vi "Exposure-Config.vi"(0 "Exposure parameters":T27, 1 "Expt State":T3, 5 "Filter options":cluster{"InvFilt":bool, "Brickwall":bool}, 7 "Sampling rate (Hz)":dbl, 9 "Buffer length (s)":dbl, 11 "error in (no error)":errorcluster, 12 "Options":T2={"Tracking"={"Tolerance (dB)"=0.25, "T (s)"=3.0}, "Seeds"={"Left"=0, "Right"=0}}) -> (2 "SPL Log":cluster{dbl, "Buffer length (s)":dbl, dbl[][]}, 3 "Runtime":T4, 4 "AO Channels":i32[](array[numeric]), 6 "stimulus":T5[](array[typedef]) {"Filter"."IIR Filter Cluster"."Forward Coefficients" format="%.4f"; "Filter"."IIR Filter Cluster"."Reverse Coefficients" format="%.4f"}, 8 "InvFilt":T1[](array[typedef]), 10 "Npts":i32, 13 "Max SPL History":dbl[][](array[numeric]), 14 "Num Buffers":i32, 15 "error out":errorcluster)   [LabVIEW 2020]
uses:
  Typedefs/Exposure Parameters.ctl
  epl-vi-lib/Signal Synthesis VIs/Controls/Stimulus Channel XCtl/Stimulus Channel Data.ctl
  epl-vi-lib/Signal Synthesis VIs/Controls/Waveform XCtl/Waveform Data.ctl
  epl-vi-lib/Signal Synthesis VIs/Controls/Waveform XCtl/Waveform Enum.ctl
  epl-vi-lib/Signal Synthesis VIs/Waveform VIs/Tone VIs/Tone Params.ctl
  epl-vi-lib/Signal Synthesis VIs/Waveform VIs/Pulse Train VIs/Pulse Train Params.ctl
  epl-vi-lib/Signal Synthesis VIs/Waveform VIs/Pulse Train VIs/Pulse Polarity.ctl
  epl-vi-lib/Signal Synthesis VIs/Waveform VIs/Pulse Train VIs/PT-Continuous State.ctl
  epl-vi-lib/Signal Synthesis VIs/Waveform VIs/Noise VIs/Noise Params.ctl
  epl-vi-lib/Signal Synthesis VIs/Waveform VIs/File VIs/StimFile-Params.ctl
  epl-vi-lib/Signal Synthesis VIs/Waveform VIs/FM Sweep VIs/FM Sweep Params.ctl
  epl-vi-lib/Signal Synthesis VIs/Waveform VIs/Chirp Train VIs/Chirp Train.ctl
  epl-vi-lib/Signal Synthesis VIs/Waveform VIs/Chirp Train VIs/Chirp Train Params.ctl
  epl-vi-lib/Signal Synthesis VIs/Waveform VIs/Complex Tone VIs/CT-Params.ctl
  epl-vi-lib/Signal Synthesis VIs/Waveform VIs/Complex Tone VIs/CT-Phase Enum.ctl
  epl-vi-lib/Signal Synthesis VIs/Waveform VIs/Complex Tone VIs/CT-Runtime Data.ctl
  epl-vi-lib/Signal Synthesis VIs/Waveform VIs/Moving Ripple VIs/Moving Ripple.ctl
  epl-vi-lib/Signal Synthesis VIs/Waveform VIs/Moving Ripple VIs/Moving Ripple.Params.ctl
  epl-vi-lib/Signal Synthesis VIs/Waveform VIs/Moving Ripple VIs/Moving Ripple.Data.ctl
  epl-vi-lib/Signal Synthesis VIs/Controls/Filter XCtl/Filter Data.ctl
  epl-vi-lib/Signal Synthesis VIs/Controls/Gate XCtl/Gate Data.ctl
  epl-vi-lib/Signal Synthesis VIs/Controls/Level XCtl/Level Data.ctl
  epl-vi-lib/Signal Synthesis VIs/Controls/Level XCtl/Level Units.ctl
  Typedefs/Exposure-Runtime Data.ctl
  CFTS Main Panel SubVIs/CFTS-Experiment State.ctl
  Typedefs/Exposure-Options.ctl
  Typedefs/Exposure-Inverse Filter Runtime.ctl
  epl-vi-lib/Connection VIs/Type Defs/Output sources.ctl
  epl-vi-lib/Connection VIs/Type Defs/Input sources.ctl
  epl-vi-lib/Utility VIs/Array Manipulation VIs/Sort and Index (I32).vi
  epl-vi-lib/Signal Synthesis VIs/Top Level VIs/Stimulus-Set Level (array).vi
  epl-vi-lib/Signal Synthesis VIs/Controls/Filter XCtl/Filter XCtl.xctl
  epl-vi-lib/Signal Synthesis VIs/Controls/Level XCtl/Level XCtl.xctl
  epl-vi-lib/Signal Synthesis VIs/Controls/Gate XCtl/Gate Control.xctl
  epl-vi-lib/Signal Synthesis VIs/Controls/Waveform XCtl/Waveform XCtl.xctl
  epl-vi-lib/Signal Synthesis VIs/Controls/Stimulus Channel XCtl/Stimulus Channel.xctl
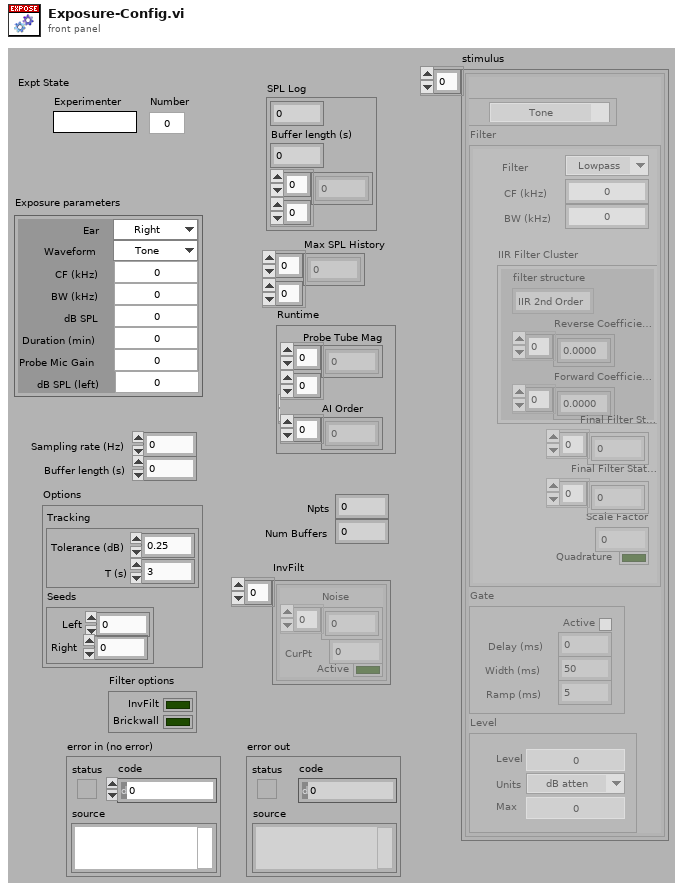
[diagram p1: front panel]
types:
  T1 = typedef "Exposure-Inverse Filter Runtime.ctl" = cluster{"Noise":dbl[], "CurPt":i32, "Active":bool}
  T2 = typedef "Exposure-Options.ctl" = cluster{"Tracking":cluster{"Tolerance (dB)":dbl, "T (s)":dbl}, "Seeds":cluster{"Left":i32, "Right":i32}}
  T3 = typedef "CFTS-Experiment State.ctl" = cluster{"Experimenter":string, "Number":u32, "Right":string, "Left":string, "Data Folder":path, "State File":path, "Version Info":string, "End Exposure Time":dbl, "Exposure Duration":string, "Run #":cluster{"CAP":i16, "ABR":i16, "DP":i16, "VsEP":i16, "MeasSeq":i16, "SubSeq":i16, "SFOAE":i16}}
  T4 = typedef "Exposure-Runtime Data.ctl" = cluster{"Probe Tube Mag":dbl[][], "AI Order":i32[]}
  T5 = typedef "Stimulus Channel.xctl/Stimulus Channel Data.ctl" = cluster{"Waveform":T6, "Filter":T23, "Gate":T24, "Level":T25}
  T6 = typedef "Waveform XCtl.xctl/Waveform Data.ctl" = cluster{"Type":T7, "Tone":T8, "Pulse Train":T9, "Noise":T12, "File":T13, "FMSweep":T14, "Chirp Train":T15, "Complex Tone":cluster{"Params":T17, "Data":T19}, "Moving Ripple":T20}
  T7 = typedef "Waveform Enum.ctl" = enum16{"OFF", "Tone", "Noise", "Pulse Train", "File", "FM Sweep", "Chirp Train", "Complex Tone", "FM Tone", "Moving Ripple"}
  T8 = typedef "Tone Params.ctl" = cluster{"Frequency (kHz)":dbl, "Last Freq":dbl, "Last Phase":dbl}
  T9 = typedef "Pulse Train Params.ctl" = cluster{"Pulse width (us)":dbl, "Pulse rate (Hz)":dbl, "Gap (ms)":dbl, "Polarity":T10, "PT State":T11, "Asynch":bool}
  T10 = typedef "Pulse Polarity.ctl" = enum16{"POS", "NEG", "POS-NEG", "NEG-POS"}
  T11 = typedef "PT-Continuous State.ctl" = cluster{"Template":dbl[], "Nperiod":i32, "Index":i32, "Pulse Rate (Hz)":dbl, "Phase (cycles)":dbl, "Noff":i32}
  T12 = typedef "Noise Params.ctl" = cluster{"InvFilt":bool, "Noise":dbl[], "CurPt":i32, "Aweight":bool, "Seed":i32, "afile":path}
  T13 = typedef "StimFile-Params.ctl" = cluster{"Filename":path, "Signal":dbl[], "Channel":i32, "stream":bool, "offset":i32, "nreps":i32, "loops":i32, "Randomize":bool, "order":i32[], "Seed":i32, "Tokens":i32}
  T14 = typedef "FM Sweep Params.ctl" = cluster{"Rate (oct/s)":dbl, "Fmin (Hz)":dbl, "Fmax (Hz)":dbl, "Ramp (ms)":dbl, "Linear":bool}
  T15 = typedef "Chirp Train.ctl" = cluster{"Params":T16, "Data":cluster{"WF":dbl[]}}
  T16 = typedef "Chirp Train Params.ctl" = cluster{"Fmin (kHz)":dbl, "Fmax (kHz)":dbl, "Compensate":bool, "Duration (ms)":dbl}
  T17 = typedef "CT-Params.ctl" = cluster{"F0 (Hz)":dbl, "Band":cluster{"Flow (Hz)":dbl, "Fhigh (Hz)":dbl}, "Phase":T18, "Min F0 (Hz)":dbl, "Max F0 (Hz)":dbl, "ContinRandPhase":bool, "Max peak factor":dbl, "Max mod depth":dbl, "MinHarmNum":i32, "MaxHarmNum":i32, "Level Mode":enum16{"per component", "overall rms"}, "% jitter":dbl}
  T18 = typedef "CT-Phase Enum.ctl" = enum16{"Cosine", "Random", "Alternating"}
  T19 = typedef "CT-Runtime Data.ctl" = cluster{"Ncomp":i32, "MinHarm":i32, "Phase":dbl[], "Amplitude":dbl[], "Npts/frame":i32, "Last F0":dbl, "Fmin":dbl, "Fmax":dbl, "Lslope":dbl, "randphase":bool, "overall rms":bool, "fmult":dbl[], "jittered":bool}
  T20 = typedef "Moving Ripple.ctl" = cluster{"Params":T21, "Data":T22}
  T21 = typedef "Moving Ripple.Params.ctl" = cluster{"Fmin":dbl, "Fmax":dbl, "Density":dbl, "Velocity":dbl, "Depth":dbl, "Phase":dbl, "Comp/oct":i32}
  T22 = typedef "Moving Ripple.Data.ctl" = cluster{"Freq":dbl[], "A":dbl[], "phase":dbl[], "Phase":dbl}
  T23 = typedef "Filter XCtl.xctl/Filter Data.ctl" = cluster{"CF (kHz)":dbl, "BW (kHz)":dbl, "IIR Filter Cluster":cluster{"filter structure":enum32{"IIR 2nd Order", "IIR 4th Order"}, "Reverse Coefficients":dbl[], "Forward Coefficients":dbl[]}, "Final Filter State":dbl[], "Scale Factor":dbl, "Final Filter State 2":dbl[], "Quadrature":bool, "Type":enum16{"Lowpass", "Highpass", "Bandpass", "Bandstop", "OFF"}}
  T24 = typedef "Gate Control.xctl/Gate Data.ctl" = cluster{"Active":bool, "Delay (ms)":dbl, "Width (ms)":dbl, "Ramp (ms)":dbl}
  T25 = typedef "Level XCtl.xctl/Level Data.ctl" = cluster{"Level":dbl, "Units":T26, "Max":dbl, "Multiplier":dbl, "Cal File":path, "Cal":cluster{"Freq (Hz)":dbl[], "Mag (dB SPL)":dbl[], "Phase (deg)":dbl[]}}
  T26 = typedef "Level Units.ctl" = enum16{"dB atten", "dB SPL", "dB re 1 Vrms", "dB V/Hz½", "mW", "dB HL", "Volts", "dB mW"}
  T27 = typedef "Exposure Parameters.ctl" = cluster{"Probe Mic Gain":dbl, "Waveform":enum16{"Tone", "Noise"}, "CF (kHz)":dbl, "BW (kHz)":dbl, "Ear":enum16{"Right", "Left", "Binaural"}, "Duration (min)":dbl, "dB SPL":dbl, "dB SPL (left)":dbl}
  T28 = typedef "Input sources.ctl" = u16
  T29 = typedef "Output sources.ctl" = u16
  T30 = cluster{"Waveform":T6, "Filter":T23, "Gate":T24, "Level":T25}[]
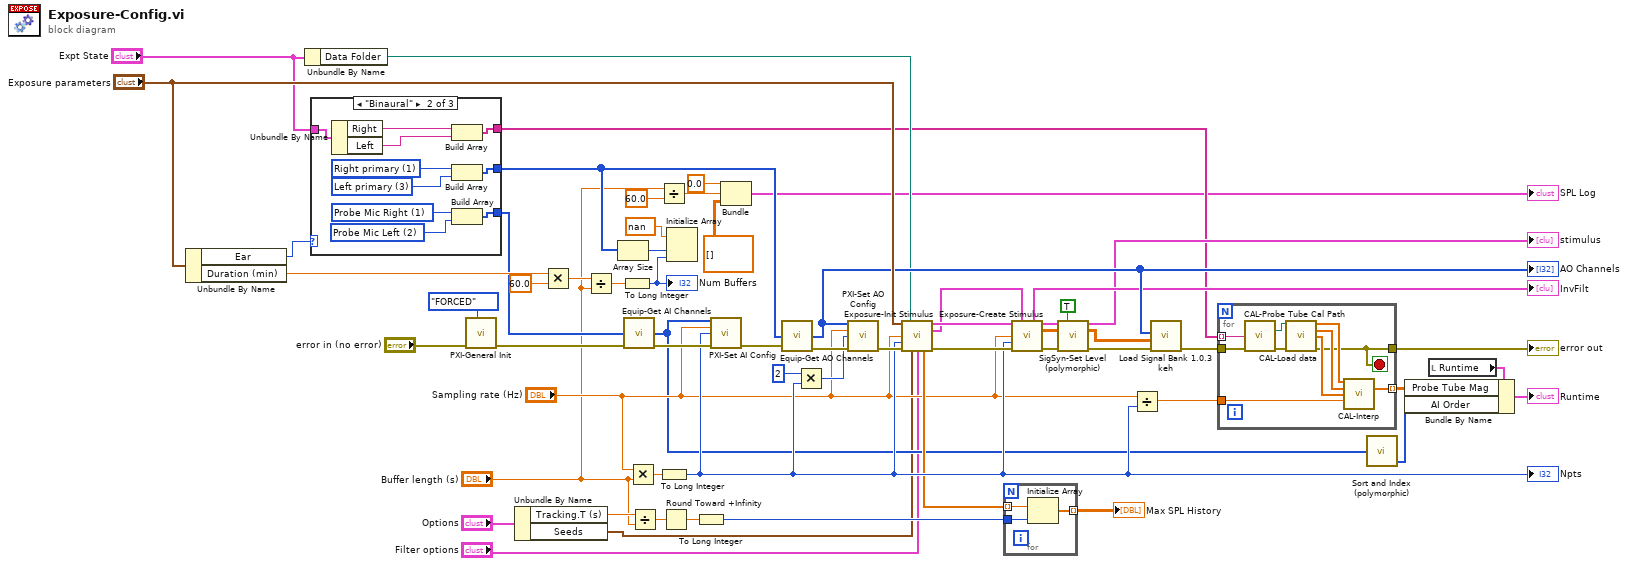
[diagram p0: block diagram]
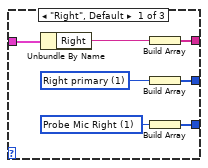
[diagram p2: hidden frame]
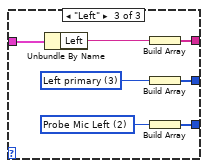
[diagram p3: hidden frame]
diagram:
  n1 = Unbundle By Name("Exposure parameters") -> ("Ear"=w25:enum16{"Right", "Left", "Binaural"}, "Duration (min)"=w49:dbl)
  n2 = Unbundle By Name("Expt State") -> ("Data Folder"=w38:path)
  n3 = case shown="\"Binaural\"" w25 {
    tunnel: [w63 w73 w80] -> w15
    tunnel: [w62 w72 w79] -> w24
    tunnel: [w64 w74 w81] -> w19
    tunnel: "Expt State" -> [w66 w76 w83]
    frame "Right", Default {
      w67 = T28 1 items=["--unused--", "Probe Mic Right", "Probe Mic Left", "Cal Mic", "ABR", "CAP Right", "CAP Left", "Startle piezo", "Temperature", "Heart rate", "Accelerometer"] ("Ring")
      w68 = T29 1 items=["--unused--", "Right primary", "Right secondary", "Left primary", "Left secondary", "Shocks", "Startle", "Background", "Shaker"] ("Ring")
      n4 = Unbundle By Name(w66) -> ("Right"=w65:string)
      n5 = Build Array(w65) -> (w64:string[])
      n6 = Build Array(w68) -> (w63:T29[])
      n7 = Build Array(w67) -> (w62:T28[])
    }
    frame "Binaural" {
      w69 = T28 2 items=["--unused--", "Probe Mic Right", "Probe Mic Left", "Cal Mic", "ABR", "CAP Right", "CAP Left", "Startle piezo", "Temperature", "Heart rate", "Accelerometer"] ("Ring")
      w70 = T29 3 items=["--unused--", "Right primary", "Right secondary", "Left primary", "Left secondary", "Shocks", "Startle", "Background", "Shaker"] ("element")
      w77 = T28 1 items=["--unused--", "Probe Mic Right", "Probe Mic Left", "Cal Mic", "ABR", "CAP Right", "CAP Left", "Startle piezo", "Temperature", "Heart rate", "Accelerometer"] ("Ring")
      w78 = T29 1 items=["--unused--", "Right primary", "Right secondary", "Left primary", "Left secondary", "Shocks", "Startle", "Background", "Shaker"] ("Ring")
      n8 = Unbundle By Name(w76) -> ("Right"=w75:string, "Left"=w71:string)
      n9 = Build Array(w75, w71) -> (w74:string[])
      n10 = Build Array(w78, w70) -> (w73:T29[])
      n11 = Build Array(w77, w69) -> (w72:T28[])
    }
    frame "Left" {
      w84 = T28 2 items=["--unused--", "Probe Mic Right", "Probe Mic Left", "Cal Mic", "ABR", "CAP Right", "CAP Left", "Startle piezo", "Temperature", "Heart rate", "Accelerometer"] ("Ring")
      w85 = T29 3 items=["--unused--", "Right primary", "Right secondary", "Left primary", "Left secondary", "Shocks", "Startle", "Background", "Shaker"] ("Ring")
      n12 = Unbundle By Name(w83) -> ("Left"=w82:string)
      n13 = Build Array(w82) -> (w81:string[])
      n14 = Build Array(w85) -> (w80:T29[])
      n15 = Build Array(w84) -> (w79:T28[])
    }
  }
  n16 = call "PXI-General Init.vi"("Double Buffer Mode"=enum32{"OFF", "ENABLED", "FORCED"}."FORCED", "error in (no error)"="error in (no error)") -> ("error out"=w58:errorcluster)  [unwired: 9 in]
  n17 = Unbundle By Name("Options") -> ("Tracking.T (s)"=w34:dbl, "Seeds"=w1:cluster{"Left":i32, "Right":i32})
  n18 = Multiply(x=w49, y=60.0) -> (x*y=w47:dbl)
  n19 = Divide(x=w47, y="Buffer length (s)") -> (x/y=w46:dbl)
  n20 = Array Size(array=w15) -> (size(s)=w16:i32)
  n21 = To Long Integer(number=w46) -> (32bit integer=w17:i32)
  "Num Buffers" <- w17
  n22 = call "Equip-Get AI Channels.vi"("Inputs"=w24, "error in (no error)"=w58) -> ("AI Channels"=w6:i32[], "error out"=w55:errorcluster)  [unwired: 12 in]
  n23 = Multiply(x="Sampling rate (Hz)", y="Buffer length (s)") -> (x*y=w57:dbl)
  n24 = Divide(x=w34, y="Buffer length (s)") -> (x/y=w33:dbl)
  n25 = Divide(x="Buffer length (s)", y=60.0) -> (x/y=w10:dbl)
  n26 = To Long Integer(number=w57) -> (32bit integer=w28:i32)
  "Npts" <- w28
  n27 = Round Toward +Infinity(x=w33) -> (ceil(x): smallest int >= x=w32:dbl)
  n28 = Initialize Array(nan ("element"), w16, w17) -> ()  [unwired: 1 out]
  n29 = To Long Integer(number=w32) -> (32bit integer=w31:i32)
  n30 = call "PXI-Set AI Config.vi"("AI Channels"=w6, "Sampling Rate (Hz)"="Sampling rate (Hz)", "Buffer Size"=w28, "error in (no error)"=w55) -> ("error out"=w52:errorcluster)  [unwired: 11 in]
  n31 = Bundle(0.0, w10, "initialized array"=dbl[][] []) -> (→"SPL Log":cluster{dbl, dbl, "initialized array":dbl[][]})  [unwired: 1 in]
  n32 = call "Equip-Get AO Channels.vi"("Outputs"=w15, "error in (no error)"=w52) -> ("AO Channels"=w42:i32[], "error out"=w54:errorcluster)  [unwired: 12 in]
  "AO Channels" <- w42
  n33 = Multiply(x=2, y=w28) -> (x*y=w53:i32)
  n34 = call "PXI-Set AO Config.vi"("AO Channels"=w42, "Sampling Rate (Hz)"="Sampling rate (Hz)", "Buffer Size"=w53, "error in (no error)"=w54) -> ("error out"=w51:errorcluster)  [unwired: 11 in]
  n35 = call "Exposure-Init Stimulus.vi"("Exposure parameters"="Exposure parameters", "Data Folder"=w38, "Sampling rate (Hz)"="Sampling rate (Hz)", "Npts"=w28, "error in (no error)"=w51, "Seeds"=w1, "Filter options"="Filter options") -> ("StimChan"=w61:T30, "InvFilt"=w30:T1[], "Max Level"=w27:dbl[], "error out"=w60:errorcluster)  [unwired: 5 in]
  n36 = for {
    tunnel: [w88] -> w36 mode=indexing
    tunnel: w31 -> [w87]
    tunnel: w27 -> [w86] mode=indexing
    n37 = Initialize Array(w86, w87) -> (w88:dbl[])
  }
  "Max SPL History" <- w36
  n38 = call "Exposure-Create Stimulus.vi"("StimChan In"=w61, "InvFilt In"=w30, "Sampling rate (Hz)"="Sampling rate (Hz)", "Npts"=w28, "error in (no error)"=w60) -> ("InvFilt Out"=→"InvFilt":T1[], "StimChan Out"=w3:T5[], "Stimulus"=w18:dbl[][], "error out"=w45:errorcluster)  [unwired: 7 in]
  n39 = call-poly "SigSyn-Set Level (polymorphic).vi"("AO Control in"=w3, "Apply multiplier? (F)"=TRUE ("Apply multiplier?"), "Waveform in"=w18, "error in (no error)"=w45) -> ("AO Control out"=→"stimulus":T30, "Waveform out"=w21:dbl[][], "error out"=w43:errorcluster)  [unwired: 6 in, 3 out]
  n40 = Divide(x="Sampling rate (Hz)", y=w28) -> (x/y=w39:dbl)
  n41 = call "Load Signal Bank 1.0.3 keh.vi"("error in (no error)"=w43, "Input array"=w21, "Active AO Array"=w42) -> ("error out"=w20:errorcluster)  [unwired: 6 in, 2 out]
  n42 = for {
    tunnel: [w89] -> w40
    tunnel: w39 -> [w95]
    tunnel: [w94] -> w37 mode=indexing
    tunnel: w20 -> [w93]
    tunnel: w19 -> [w90] mode=indexing
    stop <- w89 stop-if-true
    n43 = call "CAL-Probe Tube Cal Path.vi"("Acoustic System"=w90, "error in (no error)"=w93) -> ("Probe Tube Cal Path"=w91:path, "error out"=w92:errorcluster)  [unwired: 12 in]
    n44 = call "CAL-Load data.vi"("user path"=w91, "error in (no error)"=w92) -> ("Frequency (Hz)"=w98:dbl[], "Mag"=w97:dbl[], "Phase"=w96:dbl[], "error out"=w89:errorcluster)  [unwired: 6 in, 4 out]
    n45 = call "CAL-Interp.vi"("Frequency (Hz)"=w98, "Magnitude (dB)"=w97, "Phase (degrees)"=w96, "df (Hz)"=w95) -> ("Interp Magnitude (dB)"=w94:dbl[])  [unwired: 8 in, 3 out]
  }
  "error out" <- w40
  n46 = call-poly "Sort and Index (polymorphic).vi"("X"=w6) -> ("Index"=w5:i32[])  [unwired: 3 in, 1 out]
  n47 = local read "Runtime"() -> (w7:T4)
  n48 = Bundle By Name(cluster=w7, "Probe Tube Mag"=w37, "AI Order"=w5) -> (→"Runtime":T4)
